vi "LJUD U3RAW SetDefaults.vi"(7 "Comm Settings":T1={"Open LabJack "=TRUE, "Address"="1", "FirstFound"=TRUE}, 8 "error in (no error)":errorcluster, 11 "Handle In":i32) -> (0 "error out":errorcluster, 3 "Handle Out":i32)   [LabVIEW 2021]
panel:
  out "Write Array":u8[](array[numeric]) format="%.0x"
  out "Read Array":u8[](array[numeric]) format="%.0x"
  # "This writes to flash.  The U3 flash has a rated\nendurance of at least 20000 writes, which is\nplenty for reasonable operation, but if this\nfunction is called in a high-speed loop the\nflash could eventually be damaged."
  # "If open is false,\nthen a valid\nhandle must be\npassed in."
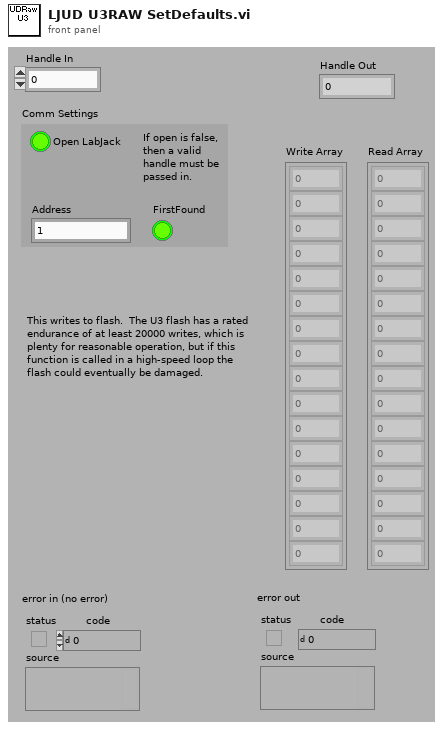
[diagram p1: front panel]
types:
  T1 = cluster{"Open LabJack ":bool, "Address":string, "FirstFound":bool}
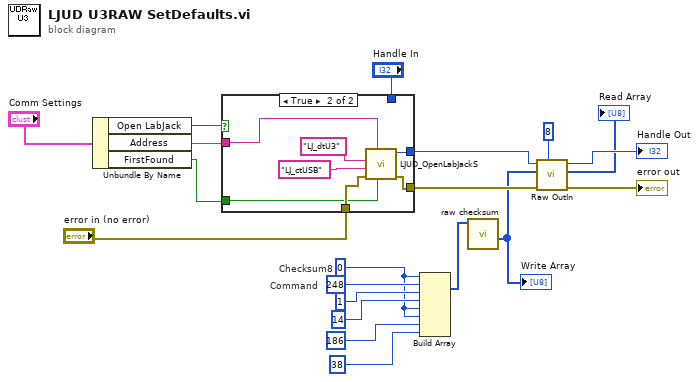
[diagram p0: block diagram]
diagram:
  w13 = u8 0  # Checksum8
  w20 = u8 248  # Command
  n1 = Unbundle By Name("Comm Settings") -> ("Open LabJack"=w11:bool, "Address"=w10:string, "FirstFound"=w9:bool)
  n2 = case shown="True" w11 {
    tunnel: w10 -> [_ w26]
    tunnel: "error in (no error)" -> [w22 w27]
    tunnel: [w22 w28] -> w7
    tunnel: [w21 w29] -> w6
    tunnel: w9 -> [_ w25]
    tunnel: "Handle In" -> [w21 _]
    frame False {
    }
    frame True {
      n3 = call "LJUD_OpenLabJackS.vi"("FirstFound"=w25, "Address"=w26, "error in"=w27, "ConnectionType"="LJ_ctUSB", "DeviceType"="LJ_dtU3") -> ("error out"=w28:errorcluster, "Handle"=w29:i32)  [unwired: 4 in, 1 out]
    }
  }
  n4 = Build Array(w13, w20, u8 1, u8 14, w13, w13, u8 186, u8 38) -> (w16:u8[])
  n5 = call "raw checksum.vi"("Array"=w16) -> ("Array Output"=w1:u8[])  [unwired: 3 in, 7 out]
  "Write Array" <- w1
  n6 = call "Raw OutIn.vi"("# of bytes to read in"=8 ("# of bytes to read"), "error in"=w7, "Raw Out"=w1, "Handle In"=w6) -> ("error out"=→"error out":errorcluster, "Raw In"=→"Read Array":u8[], "Handle Out"=→"Handle Out":i32)  [unwired: 4 in, 1 out]
